vi "Display Project Info Results.vi"(7 "Theme":bool=TRUE, 8 "error in":errorcluster, 11 "Project Info":T1[](array[typedef])) -> (0 "error out":errorcluster)   [LabVIEW 2019, in "Panther Dashboard.lvlib"]
uses:
  Panther Dashboard.lvlib
  Module Info--cluster.ctl
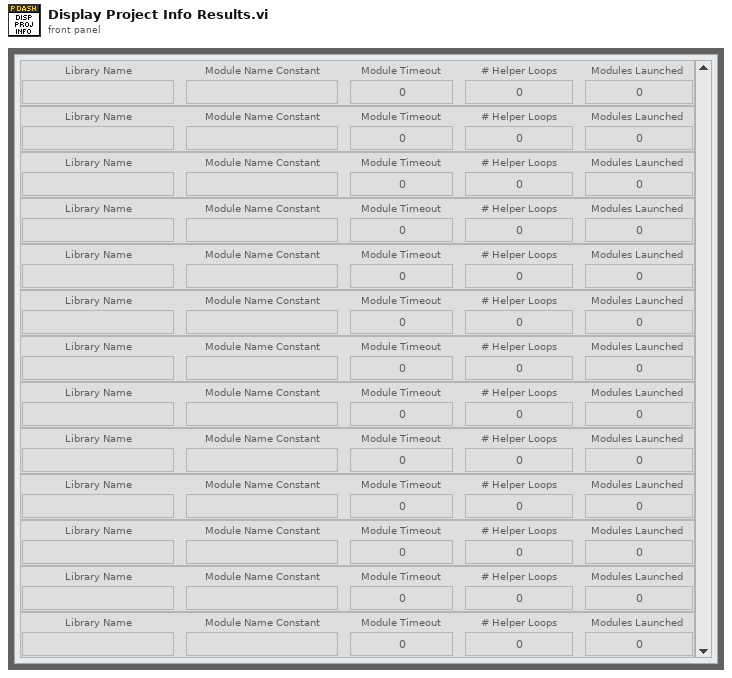
[diagram p1: front panel]
types:
  T1 = typedef "Panther Dashboard.lvlib/Module Info--cluster.ctl" = cluster{"Library Name":string, "Module Name Constant":string, "Module Timeout":i32, "# Helper Loops":i32, "Modules Launched":i32}
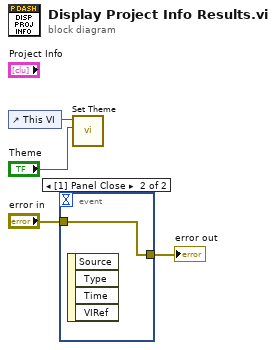
[diagram p0: block diagram]
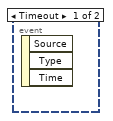
[diagram p2: hidden frame]
diagram:
  n1 = control-ref of="This VI"() -> (w1:refnum<vi>)
  n2 = event shown="[1] Panel Close" {
    selector: _ -> [_ _]
    dyn-events: _ -> [_ _]
    timeout: _ -> [_ _]
    tunnel: "error in" -> [_ w5]
    tunnel: [_ w5] -> w3
    event Timeout {
      n3 = event-data() -> ()  [unwired: 1 in, 3 out]
    }
    event Panel Close {
      n4 = event-data() -> ()  [unwired: 1 in, 4 out]
    }
  }
  "error out" <- w3
  n5 = call "Set Theme.vi"("Dark?"="Theme", "VI in"=w1) -> ()  [unwired: 10 in]
